vi "FlatToRichcif_manager_TimePair.vi"(5 "OutputClusterType":T1, 11 "InputCluster":T2) -> (3 "OutputCluster":T1)   [LabVIEW 2021, in "CIF_Launcher_server.lvlib"]
uses:
  CIF_Launcher_server.lvlib
  cif_manager_TimePair_Flat.ctl
  cif_manager_TimePair.ctl
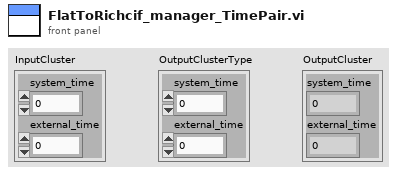
[diagram p1: front panel]
types:
  T1 = typedef "CIF_Launcher_server.lvlib/cif_manager_TimePair.ctl" = cluster{"system_time":i64, "external_time":i64}
  T2 = typedef "CIF_Launcher_server.lvlib/cif_manager_TimePair_Flat.ctl" = cluster{"system_time":i64, "external_time":i64}
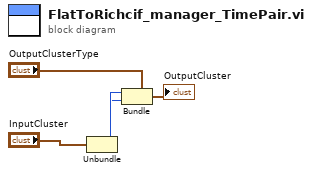
[diagram p0: block diagram]
diagram:
  n1 = Unbundle "Unbundle"("InputCluster") -> ("system_time"=w2:i64, "external_time"=w1:i64)
  n2 = Bundle "Bundle"(cluster="OutputClusterType", "system_time"=w2, "external_time"=w1) -> (→"OutputCluster":T1)
